vi "Initialise.vi"(7 "VI Ref in":refnum<vi>, 8 "error in (no error)":errorcluster, 11 "EmulatorActor in":refnum<class "EmulatorActor.lvclass">) -> (0 "error out":errorcluster, 3 "EmulatorActor out":refnum<class "EmulatorActor.lvclass">)   [LabVIEW 2019, in "EmulatorActor.lvlib" / "EmulatorActor.lvclass"]
uses:
  EmulatorActor.lvclass
  <vilib>/ActorFramework/Actor/Actor.lvclass
  DigitiserActor/DigitiserActor/DigitiserActor.lvclass
  C:/Program Files (x86)/National Instruments/LabVIEW 2019/vi.lib/ActorFramework/Actor/Actor.lvclass
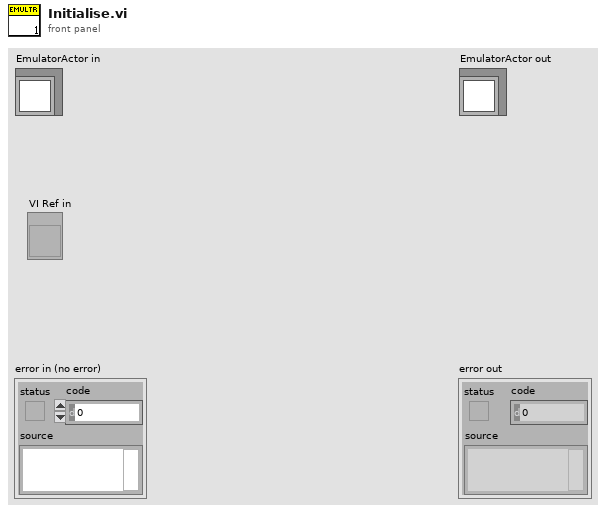
[diagram p1: front panel]
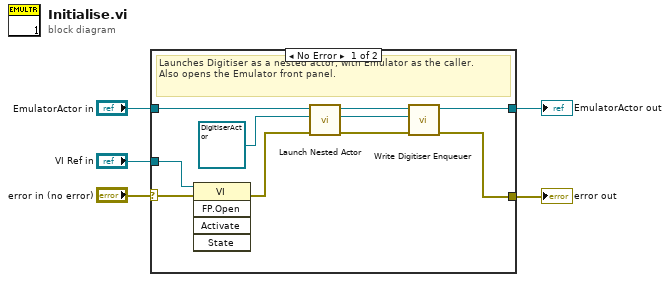
[diagram p0: block diagram]
diagram:
  n1 = case shown="No Error" "error in (no error)" {
    selector: "error in (no error)" -> [w8 w17]
    tunnel: [w13 w17] -> w4
    tunnel: [w11 w16] -> w2
    tunnel: "EmulatorActor in" -> [w6 w16]
    tunnel: "VI Ref in" -> [w9 _]
    frame No Error {
      # "Launches Digitiser as a nested actor, with Emulator as the caller.\nAlso opens the Emulator front panel."
      n2 = invoke class="VI" method="FP.Open"(reference=w9, error in=w8) -> (error out=w7:errorcluster)  [unwired: 3 in, 4 out]
      n3 = call <vilib>:"Launch Nested Actor.vi"("error in (no error)"=w7, "Nested Actor"=refnum<class "DigitiserActor.lvclass"> refnum ("DigitiserActor.lvlib:DigitiserActor.lvclass"), "Caller Actor in"=w6) -> ("error out"=w15:errorcluster, "Nested Actor's Enqueuer"=w10:refnum<class "Message Enqueuer.lvclass">, "Caller Actor out"=w12:refnum<class "Actor.lvclass">)  [unwired: 6 in]
      n4 = call "Write Digitiser Enqueuer.vi"("error in (no error)"=w15, "Actor Framework:Message Enqueuer"=w10, "EmulatorActor in"=w12) -> ("error out"=w13:errorcluster, "EmulatorActor out"=w11:refnum<class "EmulatorActor.lvclass">)  [unwired: 7 in]
    }
    frame Error {
    }
  }
  "error out" <- w4
  "EmulatorActor out" <- w2
